vi "Export Public Key.vi"(8 "error in (no error)":errorcluster, 11 "CngKey ref in":refnum<k24>) -> (0 "error out":errorcluster, 2 "Public Key":u8[](array[numeric]), 3 "CngKey ref out":refnum<k24>)   [LabVIEW 2021, in "dotNET Crypto Key Management.lvlib"]
uses:
  dotNET Crypto Key Management.lvlib
  System.Core
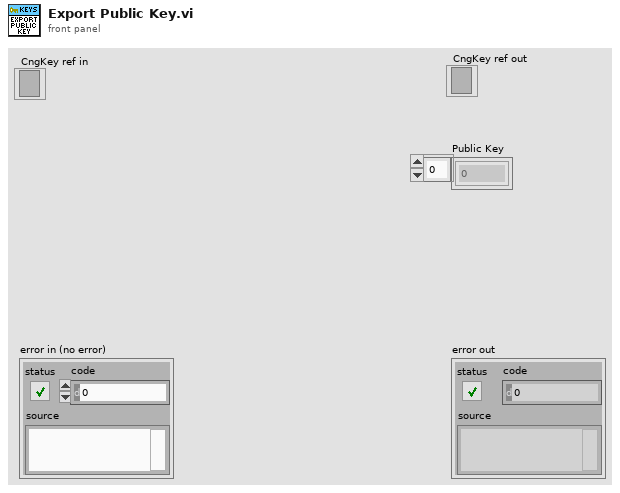
[diagram p1: front panel]
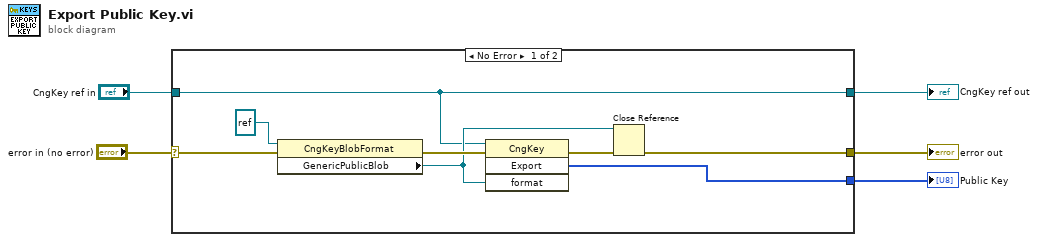
[diagram p0: block diagram]
diagram:
  n1 = case shown="No Error" "error in (no error)" {
    selector: "error in (no error)" -> [w12 w15]
    tunnel: "CngKey ref in" -> [w6 w14]
    tunnel: [w8 w15] -> w4
    tunnel: [w7 _] -> w3
    tunnel: [w6 w14] -> w1
    frame No Error {
      n2 = property class="CngKeyBlobFormat"(reference=refnum<k24> refnum ("format"), error in=w12) -> (error out=w11:errorcluster, "GenericPublicBlob"=w9:refnum<k24>)  [unwired: 1 out]
      n3 = invoke class="CngKey" method="Export"(reference=w6, error in=w11, "format"=w9) -> (error out=w10:errorcluster, "Export"=w7:u8[])  [unwired: 1 in, 2 out]
      n4 = Close Reference(reference=w9, error in (no error)=w10) -> (error out=w8:errorcluster)
    }
    frame Error {
    }
  }
  "error out" <- w4
  "Public Key" <- w3
  "CngKey ref out" <- w1
